vi "PvgeneratorOP150_2.vi"(8 "errin":errorcluster, 9 "BDD":T1, 10 "network":path, 11 "path in":path) -> (0 "sortie d'erreur":errorcluster caption="errout", 1 "network out":path, 2 "tout bon":bool, 3 "Chaîne":string)   [LabVIEW 2020]
uses:
  OP150/VG/IS30%.vi
  OP150/VG/PN.vi
  <vilib>/Utility/config.llb/NI_LVConfig.lvlib
  OP150 - Copie/SubVI/VG_HYDRAU.vi
panel:
  out "nombre de remplacements":i32
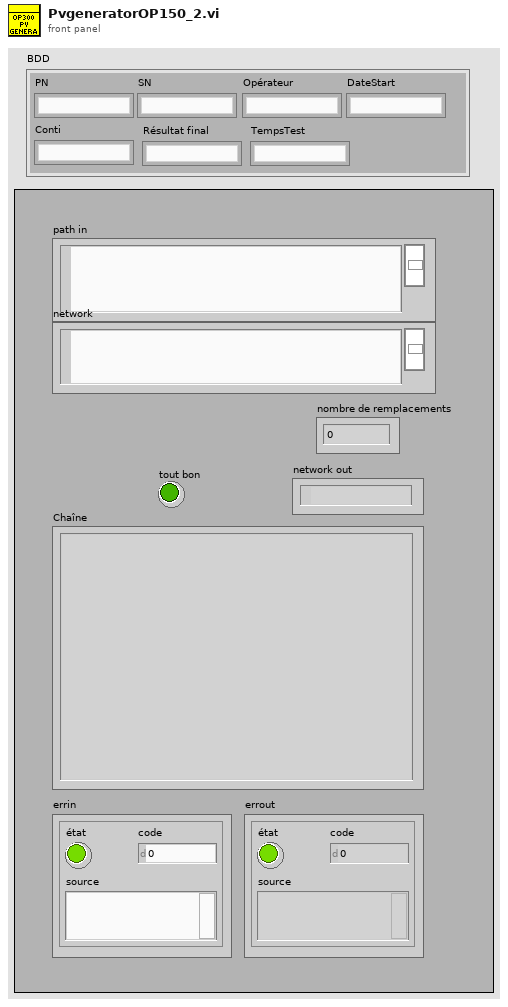
[diagram p1: front panel]
types:
  T1 = cluster{"PN":string, "Opérateur":string, "Conti":string, "Résultat final":string, "SN":string, "DateStart":string, "TempsTest":string}
  T2 = enum16{"open", "replace", "create", "open or create", "replace or create", "replace or create with confirmation"}
  T3 = typedef "NI_LVConfig.lvlib/Config Data RefNum.ctl" = refnum<k1>
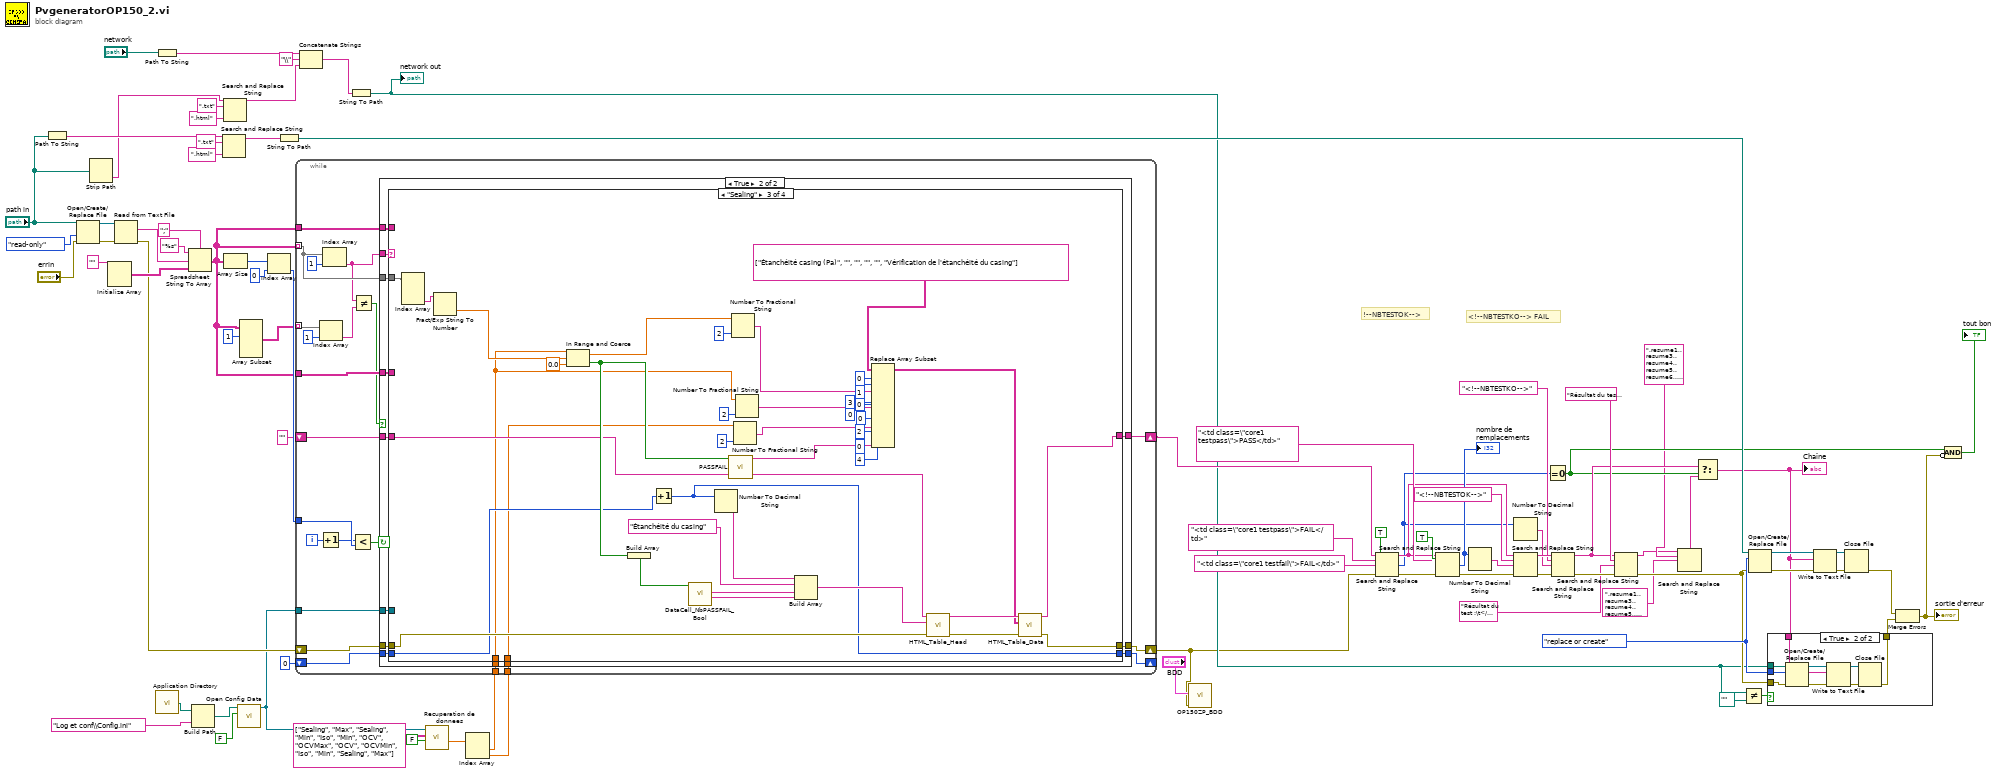
[diagram p0: block diagram]
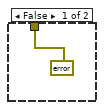
[diagram p2: hidden frame]
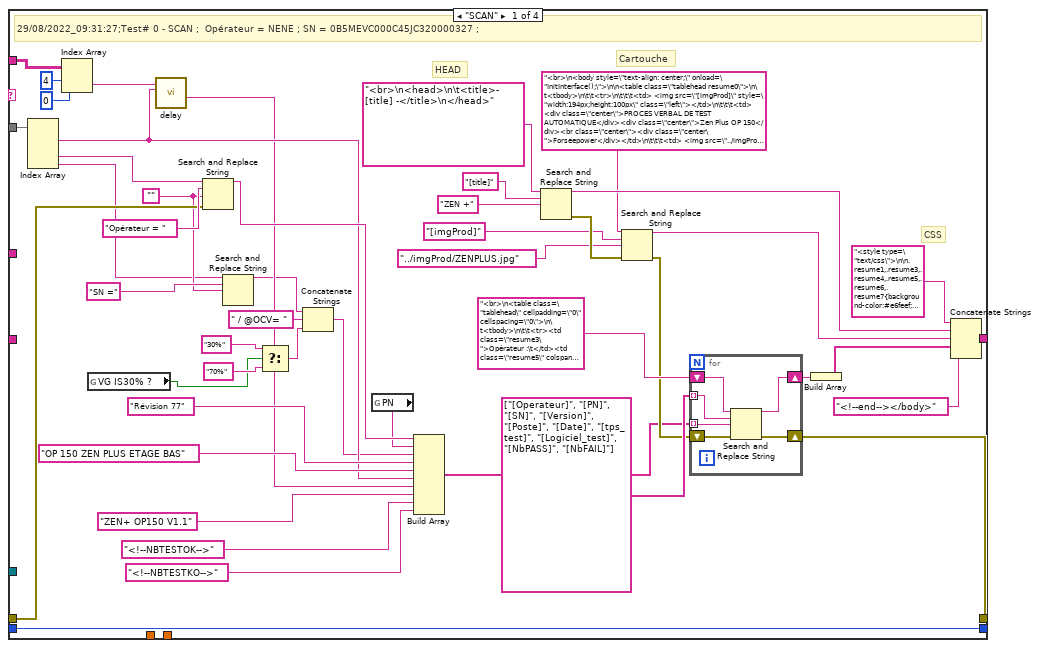
[diagram p4: hidden frame]
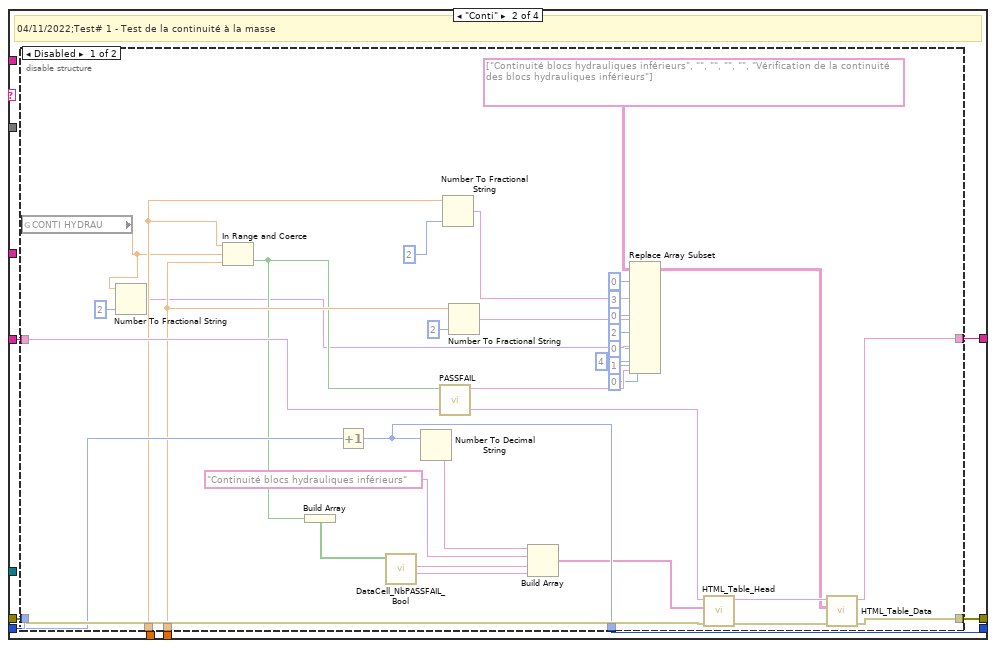
[diagram p5: hidden frame]
diagram:
  w44 = T2."replace or create" ("opération (0 : open)")
  # "<!--NBTESTKO--> FAIL"
  # "!--NBTESTOK-->"
  n1 = Path To String(path="path in") -> (string=w65:string)
  n2 = Open/Create/Replace File(file path (use dialog)="path in", error in="errin", access (0:read/write)=enum16{"read/write", "read-only", "write-only"}."read-only" ("accès (0 : read/write)")) -> (refnum out=w66:refnum<file>, error out=w83:errorcluster)  [unwired: 3 in, 1 out]
  n3 = Strip Path(path="path in") -> (name=w25:string)  [unwired: 1 out]
  n4 = Initialize Array("") -> (w81:string[][])  [unwired: 2 in]
  n5 = Read from Text File(file (use dialog)=w66, error in=w83) -> (text=w79:string, error out=w71:errorcluster)  [unwired: 2 in, 2 out]
  n6 = Path To String(path="network") -> (string=w24:string)
  n7 = call <vilib>:"Application Directory.vi"() -> ("Application Directory"=w16:path)
  n8 = Spreadsheet String To Array(delimiter (Tab)=";" ("séparateur (Tabulation)"), format string="%s" ("chaîne de format"), spreadsheet string=w79, array type (2D Dbl)=w81) -> (array=w6:string[][])
  n9 = Build Path(base path=w16, name or relative path="Log et conf\\Config.ini") -> (appended path=w19:path)
  n10 = Search and Replace String(input string=w65, search string=".txt" ("chaîne recherchée"), replace string=".html" ("chaîne de remplacement (\"\")")) -> (result string=w62:string)  [unwired: 5 in, 3 out]
  n11 = Search and Replace String(input string=w25, search string=".txt" ("chaîne recherchée"), replace string=".html" ("chaîne de remplacement (\"\")")) -> (result string=w22:string)  [unwired: 5 in, 3 out]
  n12 = Array Size(array=w6) -> (size(s)=w77:i32[])
  n13 = call <vilib>:"Open Config Data.vi"("create file if necessary (T)"=FALSE, "configuration file path"=w19) -> ("refnum"=w3:T3)  [unwired: 7 in, 2 out]
  n14 = Array Subset(array=w6, index (row)=1 ("indice")) -> (w4:string[][])  [unwired: 3 in]
  n15 = Index Array(array=w77, index=0 ("indice")) -> (element=w75:i32)
  n16 = String To Path(string=w62) -> (path=w61:path)
  n17 = Concatenate Strings(w24, "\\" ("chaîne"), w22) -> (w21:string)
  n18 = String To Path(string=w21) -> (path=w27:path)
  "network out" <- w27
  n19 = call "Recuperation de donnees.vi"("Est-ce un string?"=FALSE, "Array in"=string[][] [["Sealing", "Max"], ["Sealing", "Min"], ["Iso", "Min"], ["OCV", "OCVMax"], ["OCV", "OCVMin"], ["Iso", "Min"], ["Sealing", "Max"]], "Refnum in"=w3) -> ("Array"=w13:dbl[])  [unwired: 7 in, 1 out]
  n20 = Index Array(array=w13) -> (element #1=w12:dbl, element #2=w11:dbl)  [unwired: 2 in]
  n21 = while {
    tunnel: w75 -> [w105]
    tunnel: w6 -> [w102] mode=indexing
    shift-right: [w101] -> w1
    shift-left: w71 -> [w100]
    shift-right: [w94] -> w60
    shift-left: "" -> [w99]
    shift-right: [w97] -> _
    shift-left: 0 -> [w98]
    tunnel: w6 -> [w96]
    tunnel: w12 -> [w93]
    tunnel: w11 -> [w92]
    tunnel: w6 -> [w91]
    tunnel: w4 -> [w89] mode=indexing
    tunnel: w3 -> [w85]
    i -> [w106]
    stop <- w104 continue-if-true
    n22 = Index Array(array=w89, index=1 ("indice")) -> (element=w88:string)
    n23 = Increment(x=w106) -> (x+1=w95:i32)
    n24 = Index Array(array=w102, index=1 ("indice")) -> (element=w87:string)
    n25 = Less?(x=w95, y=w105) -> (x < y?=w104:bool)
    n26 = Not Equal?(x=w87, y=w88) -> (x != y?=w86:bool)
    n27 = case shown="True" w86 {
      tunnel: w102 -> [_ w122]
      tunnel: [w108 w121] -> w101
      tunnel: w100 -> [w108 w120]
      tunnel: w99 -> [w109 w119]
      tunnel: w98 -> [w107 w118]
      tunnel: [w107 w117] -> w97
      tunnel: w96 -> [_ w116]
      tunnel: [w109 w115] -> w94
      tunnel: w87 -> [_ w114]
      tunnel: w93 -> [_ w113]
      tunnel: w92 -> [_ w112]
      tunnel: w91 -> [_ w111]
      tunnel: w85 -> [_ w110]
      frame False {
      }
      frame True {
        n28 = case shown="\"Sealing\"" w114 {
          tunnel: w120 -> [w167 w183 w240 w260]
          tunnel: w122 -> [w169 _ w221 _]
          tunnel: [w146 w182 w239 w260] -> w121
          tunnel: w119 -> [_ w181 w235 w258]
          tunnel: w118 -> [w145 w180 w238 w259]
          tunnel: [w145 w179 w237 w259] -> w117
          tunnel: w116 -> [_ _ _ _]
          tunnel: [w144 w178 w236 w258] -> w115
          tunnel: w113 -> [_ w177 w232 _]
          tunnel: w112 -> [_ w176 w228 _]
          tunnel: w111 -> [w137 _ _ _]
          tunnel: w110 -> [_ _ _ _]
          frame "SCAN" {
            w140 = ""
            # "Cartouche"
            # "HEAD"
            # "CSS"
            # "29/08/2022_09:31:27;Test# 0 - SCAN ;  Opérateur = NENE ; SN = 0B5MEVC000C45JC320000327 ;"
            n29 = Index Array(array=w169) -> (element #1=w133:string, element #3=w143:string, element #4=w138:string)  [unwired: 4 in, 1 out]
            n30 = Index Array(array=w137, index (row)=4, index (col)=0 ("disabled index (col)")) -> (element=w134:string)
            n31 = global read "IS30%.vi" "VG IS30% ?"() -> (w124:bool)
            n32 = call "delay.vi"("String"=w133, "String 2"=w134) -> ("Delay calculé"=w132:string)  [unwired: 9 in]
            n33 = Search and Replace String(input string=w143, search string="Opérateur = " ("chaîne recherchée"), replace string=w140, error in=w167) -> (result string=w142:string)  [unwired: 4 in, 3 out]
            n34 = Search and Replace String(input string=w138, search string="SN =" ("chaîne recherchée"), replace string=w140) -> (result string=w130:string)  [unwired: 5 in, 3 out]
            n35 = Select(t="30%" ("y"), s=w124, f="70%" ("y")) -> (s? t:f=w127:string)
            n36 = Concatenate Strings(w130, " / @OCV= " ("chaîne"), w127) -> (w129:string)
            n37 = global read "PN.vi" "PN"() -> (w123:string)
            n38 = Build Array(w142, w123, w129, "Révision 77" ("element"), "OP 150 ZEN PLUS ETAGE BAS" ("chaîne"), w133, w132, "ZEN+ OP150 V1.1" ("chaîne"), "<!--NBTESTOK-->" ("chaîne"), "<!--NBTESTKO-->" ("chaîne")) -> (w147:string[])
            n39 = Search and Replace String(input string="<br>\n<head>\n\t<title>- [title] -</title>\n</head>", search string="[title]" ("chaîne recherchée"), replace string="ZEN +" ("Title")) -> (result string=w163:string, error out=w162:errorcluster)  [unwired: 5 in, 2 out]
            n40 = Search and Replace String(input string="<br>\n<body style=\"text-align: center;\" onload=\"InitInterface();\">\n\n<table class=\"tablehead resume0\">\n\t<tbody>\n\t\t<tr>\n\t\t\t<td> <img src=\"[imgProd]\" style=\"width:194px;height:100px\" class=\"left\"></td>\n\t\t\t<td> <div class=\"center\">PROCES VERBAL DE TEST AUTOMATIQUE</div><div class=\"center\">Zen Plus OP 150</div><br class=\"center\"><div class=\"center\">Forseepower</div></td>\n\t\t\t<td> <img src=\"../imgProd/LOGO FORSEE.png\" style=\"width:auto;height:auto\"  class=\"right\"></td>\n\t\t</tr>\n\t</tbody>\n</table>", search string="[imgProd]", replace string="../imgProd/ZENPLUS.jpg" ("imgProd"), error in=w162) -> (result string=w160:string, error out=w157:errorcluster)  [unwired: 4 in, 2 out]
            n41 = for {
              shift-right: [w174] -> w156
              shift-left: "<br>\n<table class=\"tablehead\" cellpadding=\"0\" cellspacing=\"0\">\n\t<tbody>\n\t\t<tr><td class=\"resume3\">Opérateur :\t</td><td class=\"resume5\" colspan=\"3\">[Operateur]</td></tr>\n\t\t<tr><td class=\"resume3\">PN : </td><td class=\"resume5\" colspan=\"3\">[PN]</td></tr>\n\t\t<tr><td class=\"resume3\">SN : </td><td class=\"resume5\" colspan=\"3\">[SN]</td></tr>\n\t\t<tr><td class=\"resume3\">Version : </td><td class=\"resume5\" colspan=\"3\">[Version]</td></tr>\n\t\t<tr><td class=\"resume3\">Poste : </td><td class=\"resume5\" colspan=\"3\">[Poste]</td></tr>\t\t\n\t\t<tr><td class=\"resume3\">Date du test : </td><td class=\"resume5\" colspan=\"3\">[Date]</td></tr>\n\t\t<tr><td class=\"resume3\">Temps de test : </td><td class=\"resume5\" colspan=\"3\">[tps_test]</td></tr>\n\t\t<tr><td class=\"resume3\">Logiciel de test :\t</td><td class=\"resume5\" colspan=\"3\">[Logiciel_test]</td></tr>\n\t\t<tr><td class=\"resume3\">Résultat du test :\t</td><td class=\"resume5\" colspan=\"3\"><div><span style=\"float:left\" id=\"result\"><font size = \"5pt\" color=\"green\"><b>CONFORME</b></font><b><font size = \"5pt\"> ( </font><font size = \"5pt\" color=\"green\">[NbPASS] PASS </font>  <font size = \"5pt\"> / </font><font size = \"5pt\" color=\"red\">[NbFAIL] FAIL</font> <font size = \"5pt\"> ) </font></b></span></div></td></tr>\n\t</tbody>\n</table>" -> [w175]
              tunnel: string[] ["[Operateur]", "[PN]", "[SN]", "[Version]", "[Poste]", "[Date]", "[tps_test]", "[Logiciel_test]", "[NbPASS]", "[NbFAIL]"] -> [w171] mode=indexing
              tunnel: w147 -> [w170] mode=indexing
              shift-right: [w172] -> w146
              shift-left: w157 -> [w173]
              n42 = Search and Replace String(input string=w175, search string=w171, replace string=w170, error in=w173) -> (result string=w174:string, error out=w172:errorcluster)  [unwired: 4 in, 2 out]
            }
            n43 = Build Array(w156) -> (w155:string[])
            n44 = Concatenate Strings("<style type=\"text/css\">\n\n.resume1,.resume3,.resume4,.resume5,.resume6,.resume7{background-color:#e6feef;padding:7px;border:1px solid black;}\n.resume0{border:1px solid black;background-color:#e6feef;font-weight: bold;padding:0px;text-align: center;}\n.resume1{width:350px;text-align:right;font-weight:bold;}\n.resume3{width:350px;text-align:right;border-top:0px solid black;font-weight:bold;}\n.resume4{border-left:0px solid black;width:290px;}\n.resume5{width:290px;border-left:0px solid black;border-top:0px solid black;}\n.resume6{border-left:0px solid black;width:60px;}\n.resume7{border-left:0px solid black;border-top:0px solid black;width:60px;}\n.title1{text-align: left;background-color:#e6f4fe;padding:10px;border:1px solid #101010;}\n.title2{width: 30px;text-align: center;background-color:#e6f4fe;padding:1px;border:1px solid #101010;border-left:0px solid black;font-weight: bold;}\n.title2 a:link{text-decoration:none;}\n.entete0,.entete1,.entete2,.time2{text-align: center;background-color:#feeec9;padding:7px;border:1px solid black;font-weight: bold;}\n.entete0{width:45px;border-right:0px solid black;}\n.entete1{width:505px;}\n.entete2{width:95px;border-right:0px solid black;}\n.time2{border-left:0px solid black;width:145px;font-size:11px;}\n.core0,.core1,.core2,.core3,.core4,.time{text-align: center;background-color:#fafed3;padding:7px;border:1px solid black;}\n.core0, .core1,.core3,.core4{width:95px;border-top:0px solid black;border-right:0px solid black;}\n.core0{width:45px;}\n.core2{border-top:0px solid black;width:505px;}\n.core3{width:200px;}\n.core4{width:300px;}\n.time{width:145px;border-top:0px solid black;border-left:0px solid black;font-size:11px;}\n.false .core0,.false .core1,.false .core2,.false .core3,.false .core4,.false .time{background-color:#f4f4f4;}\n.false .entete0,.false .entete1,.false .entete2,.false .time2{background-color:#dadada;}\n.false .title1,.false .title2,.false .resultentete .testpass,.false .resultentete .testfail,.false .resultentete .testtime{background-color:#c5cac9;color: blue;}\n.false .title2 a:link{text-decoration:none;color: blue;}\n.comment1,.comment2,.time3{width: 890px;background-color:#e9e8e9;padding:7px;border:1px solid black;border-top:0px solid black;text-align:left;}\n.comment2{border-right:0px solid black;width: 45px;text-align: center;}\n.time3{width: 145px;border-left:0px solid black;font-size:11px;}\n.fixe1{background: -moz-linear-gradient(center top , #101010 10%, #555555 80%) repeat scroll 0 0 transparent;background: -webkit-gradient(linear, left top, left bottom, from(#101010), to(#555555));border:2px solid orange;position : fixed;margin-top:20px;display:none;overflow-y:scroll;max-height:350px;text-shadow: 0px 0px 0 #333333;text-align:left;font-size:10px;padding:10px;margin-left:-162px;border-radius: 15px 15px 15px 15px;}\n.menufixe, .menufixelock{background: -moz-linear-gradient(center top , #101010 80%, transparent 20%) repeat scroll 0 0 transparent;background: -webkit-gradient(linear, left top, left bottom, from(#101010), color-stop(0.65, #101010), to(transparent)) repeat scroll 0 0 transparent;margin: -52px 0px 0px -9px;width:100%;position:fixed;height:55px;-moz-transition: margin 1s;-webkit-transition: margin 1s;}\n.menufixelock, .menufixe:hover{margin: -9px 0px 0px -9px;}\n.lockmenu, .separation,.separationmenu{text-align:center;background: -moz-linear-gradient(center top , #555555 10%, #111111 80%) repeat scroll 0 0 transparent;background: -webkit-gradient(linear, left top, left bottom, from(#555555), to(#111111));border: 1px solid white;border-radius: 10px 10px 10px 10px;box-shadow: 0 -1px 1px #555555 inset;color: #999999;font-weight: bold;width: 100px;padding: 2px;text-decoration: none;}\n.tablehead{width: 1000px;font-family: Verdana;font-size: 12px;margin-left: auto;margin-right: auto;}\n.tablenull{font-family: Verdana;font-size: 11px;margin-left: auto;margin-right: auto;}\n.separationmenu:hover div{display: inline;}\n.lockmenu:hover, .separation:hover,.separationmenu:hover{border: 1px solid orange;cursor:pointer;}\n.lockmenu:hover{border: 1px solid red;cursor:pointer;}\n.separationright{padding:10px;}\ndiv a:link{text-decoration:none;color:#cbcbcb;}\ndiv a:hover{text-decoration:underline;color:#cbcbcb;}\nspan a:link{text-decoration:none;color:#cbcbcb;}\nspan a:hover{text-decoration:none;color:#cbcbcb;}\n.false{color: blue;}\n.testpass{color: green;font-weight: bold;}\n.testfail{color: red;font-weight: bold;}\n.testtime{color: blue;font-weight: bold;}\n.resultentete{font-weight: bold;font-size: 11px;min-width: 200px;text-align:right;}\n.infohard{border: 1px solid black;background-color: white;text-align: center;width: 16px;height: 16px;border-radius: 5px;font-weight: bold;box-shadow: 0 -1px 2px #555555 inset;}\n.infohard:hover{background-color:#feeec9;cursor:pointer;}\n.footerhard{padding-top:30px;}\n.confighard{font-size:10px;width:110px;}\n.circlemain{margin-left:auto;margin-right:auto;}\n.circletext,.circleform{padding-top: 3px;text-align:center;font-size: 10px;width:200px;}\n.circleform{padding-bottom: 3px;padding-top: 1px;}\n.circle{border: 1px solid black;border-collapse: collapse;border-radius: 15px;box-shadow: 1px 1px 0 #505050;height: 15px;width: 15px;display:inline-block;}\n.bookmarkon, .bookmarkoff{background-color: yellow;border: 1px solid black;border-collapse: collapse;border-radius: 10px 10px 10px 10px;box-shadow: 1px 1px 0 #505050;height: 12px;width: 12px;position: absolute;margin-left:22px;cursor: help;}\n.bookmarkoff{background-color: transparent;border: 1px solid #CECECE;box-shadow: none;cursor: copy;}\n.false .bookmarkoff{background-color: transparent;border: 1px solid #E6E1E1;box-shadow: none;cursor: copy;}\n.bookmarkmaster{height: 15px;margin-right: 12px;width: 60px;}\n.bookmarkmaster:hover .bookmarkprev,.bookmarkmaster:hover .bookmarksuiv{display:block;}\n.bookmarkprev, .bookmarksuiv {cursor: pointer;font-size: 25px;font-weight: bold;margin-top: -10px;position: absolute;display:none;}\n.bookmarkprev{margin-left: 2px;}\n.bookmarksuiv{margin-left: 43px;}\n.plus, .moins{background-color: #F4F4F4;border: 1px solid #848484;border-radius: 20px;color: #848484;font-family: arial;font-size: 16px;font-weight: bold;height: 20px;margin-left: 4px;text-align: center;width: 20px;}\n.moins{font-size: 15px;}\n.plus:hover, .moins:hover{background-color: #DADADA;border: 1px solid black;color: black;cursor:pointer;}\n.backtothetop {position: fixed; right: 50%; margin-right: -555px; bottom: 10px; font-size: 35px; font-weight: bold; border: 1px solid #7D7B91; width: 40px; height: 40px; line-height:52px; text-align: center;border-radius: 8px; opacity: 0.25; background-color: #F5F5F5; color:#7D7B91;}\n.backtothetop:hover {opacity: 1; cursor:pointer;}\n.libversion {font-size: 8px;font-weight: normal;padding-right: 10px;text-align: right;}\n.lockmenu {width: 18px;font-size: 12px;}\n.left {display: block; margin-left: 1px;margin-right: auto;}\n.right {display: block; margin-right: 1px;margin-left: auto;}\n.center {display: block; margin-left: auto;margin-right: auto;}\n\n</style>", w163, w160, w155, "<!--end--></body>") -> (w144:string)
          }
          frame "Conti" {
            # "04/11/2022;Test# 1 - Test de la continuité à la masse"
            n45 = disable-structure shown="Disabled" {
              disable-tunnel: w183 -> [w218 _]
              disable-tunnel: [w217 _] -> w182
              disable-tunnel: w181 -> [w216 _]
              disable-tunnel: w180 -> [w215 _]
              disable-tunnel: [w214 _] -> w179
              disable-tunnel: [w213 _] -> w178
              disable-tunnel: w177 -> [w212 _]
              disable-tunnel: w176 -> [w211 _]
              frame Disabled {
                n46 = global read "VG_HYDRAU.vi" "CONTI HYDRAU"() -> (w197:dbl)
                n47 = Number To Fractional String(number=w197, precision (6)=i16 2 ("précision (6)")) -> (F-format string=w189:string)  [unwired: 2 in]
                n48 = In Range and Coerce(upper limit=w212, x=w197, lower limit=w211) -> (In Range?=w198:bool)  [unwired: 1 out]
                n49 = Build Array(w198) -> (w203:bool[])
                n50 = Increment(x=w215) -> (x+1=w214:i32)
                n51 = call "DataCell_NbPASSFAIL_Bool.vi"("Tableau en entrée"=w203) -> ("Chaîne"=w201:string, "Chaîne 2"=w202:string)  [unwired: 8 in, 1 out]
                n52 = Number To Decimal String(number=w214) -> (decimal integer string=w206:string)  [unwired: 1 in]
                n53 = call "PASSFAIL.vi"("E"=w198) -> ("S"=w186:string)  [unwired: 10 in]
                n54 = Number To Fractional String(number=w212, precision (6)=i16 2) -> (F-format string=w195:string)  [unwired: 2 in]
                n55 = Number To Fractional String(number=w211, precision (6)=i16 2) -> (F-format string=w192:string)  [unwired: 2 in]
                n56 = Build Array(w206, "Continuité blocs hydrauliques inférieurs" ("élément"), w202, w201) -> (w209:string[])
                n57 = Replace Array Subset(array=string[][] [["Continuité blocs hydrauliques inférieurs", "", "", "", "", "Vérification de la continuité des blocs hydrauliques inférieurs"]] ("Tableau"), new element #1=w195, index (row) #1=0 ("indice (ligne)"), index (col) #1=3 ("indice désactivé (col)"), new element #2=w192, index (row) #2=0 ("indice (ligne)"), index (col) #2=2 ("indice désactivé (col)"), new element #3=w189, index (row) #3=0 ("indice (ligne)"), index (col) #3=1 ("indice désactivé (col)"), new element #4=w186, index (row) #4=0 ("indice (ligne)"), index (col) #4=4 ("indice désactivé (col)")) -> (w204:string[][])
                n58 = call "HTML_Table_Head.vi"("entrée d'erreur (pas d'erreur)"=w218, "Tableau"=w209, "chaîne en entrée"=w216) -> ("sortie d'erreur"=w208:errorcluster, "result string"=w207:string)  [unwired: 7 in]
                n59 = call "HTML_Table_Data.vi"("entrée d'erreur (pas d'erreur)"=w208, "Tableau"=w204, "chaîne en entrée"=w207) -> ("sortie d'erreur"=w217:errorcluster, "result string"=w213:string)  [unwired: 7 in]
              }
              frame Enabled {
              }
            }
          }
          frame "Sealing" {
            (unwired) 0 ("index (row)")
            n60 = Index Array(array=w221) -> (element #3=w220:string)  [unwired: 3 in, 2 out]
            n61 = Fract/Exp String To Number(string=w220) -> (number=w233:dbl)  [unwired: 3 in, 1 out]
            n62 = In Range and Coerce(upper limit=w232, x=w233, lower limit=0.0) -> (coerced(x)=w234:dbl, In Range?=w246:bool)
            n63 = Build Array(w246) -> (w251:bool[])
            n64 = Increment(x=w238) -> (x+1=w237:i32)
            n65 = call "DataCell_NbPASSFAIL_Bool.vi"("Tableau en entrée"=w251) -> ("Chaîne"=w249:string, "Chaîne 2"=w250:string)  [unwired: 8 in, 1 out]
            n66 = Number To Decimal String(number=w237) -> (decimal integer string=w254:string)  [unwired: 1 in]
            n67 = call "PASSFAIL.vi"("E"=w246) -> ("S"=w224:string)  [unwired: 10 in]
            n68 = Number To Fractional String(number=w234, precision (6)=i16 2) -> (F-format string=w245:string)  [unwired: 2 in]
            n69 = Number To Fractional String(number=w228, precision (6)=i16 2) -> (F-format string=w227:string)  [unwired: 2 in]
            n70 = Number To Fractional String(number=w232, precision (6)=i16 2) -> (F-format string=w242:string)  [unwired: 2 in]
            n71 = Build Array(w254, "Étanchéité du casing" ("élément"), w250, w249) -> (w257:string[])
            n72 = Replace Array Subset(array=string[][] [["Étanchéité casing (Pa)", "", "", "", "", "Vérification de l'étanchéité du casing"]] ("Tableau"), new element #1=w245, index (row) #1=0 ("indice (ligne)"), index (col) #1=1 ("indice désactivé (col)"), new element #2=w242, index (row) #2=0 ("index (row)"), index (col) #2=3 ("disabled index (col)"), new element #3=w227, index (row) #3=0 ("index (row)"), index (col) #3=2 ("disabled index (col)"), new element #4=w224, index (row) #4=0 ("index (row)"), index (col) #4=4 ("disabled index (col)")) -> (w252:string[][])
            n73 = call "HTML_Table_Head.vi"("entrée d'erreur (pas d'erreur)"=w240, "Tableau"=w257, "chaîne en entrée"=w235) -> ("sortie d'erreur"=w256:errorcluster, "result string"=w255:string)  [unwired: 7 in]
            n74 = call "HTML_Table_Data.vi"("entrée d'erreur (pas d'erreur)"=w256, "Tableau"=w252, "chaîne en entrée"=w255) -> ("sortie d'erreur"=w239:errorcluster, "result string"=w236:string)  [unwired: 7 in]
          }
          frame "NULL", Default {
            # "NULL"
          }
        }
      }
    }
  }
  n75 = call "OP150ZP_BDD.vi"("errin"=w1, "DATA IN"="BDD") -> ()  [unwired: 9 in, 1 out]
  n76 = Search and Replace String(replace all?=TRUE ("tout remplacer ? (F)"), input string=w60, search string="<td class=\"core1 testpass\">FAIL</td>" ("chaîne recherchée"), replace string="<td class=\"core1 testfail\">FAIL</td>" ("chaîne de remplacement (\"\")"), error in=w1) -> (result string=w45:string, number of replacements=w40:i32, error out=w56:errorcluster)  [unwired: 3 in, 1 out]
  n77 = Search and Replace String(replace all?=TRUE ("tout remplacer ? (F)"), input string=w45, search string="<td class=\"core1 testpass\">PASS</td>" ("chaîne recherchée"), error in=w56) -> (number of replacements=w48:i32, error out=w52:errorcluster)  [unwired: 4 in, 2 out]
  "nombre de remplacements" <- w48
  n78 = Number To Decimal String(number=w48) -> (decimal integer string=w47:string)  [unwired: 1 in]
  n79 = Number To Decimal String(number=w40) -> (decimal integer string=w46:string)  [unwired: 1 in]
  n80 = Search and Replace String(input string=w45, search string="<!--NBTESTOK-->" ("chaîne recherchée"), replace string=w47, error in=w52) -> (result string=w53:string, error out=w51:errorcluster)  [unwired: 4 in, 2 out]
  n81 = Equal To 0?(x=w40) -> (x = 0?=w32:bool)
  n82 = Search and Replace String(input string=w53, search string="<!--NBTESTKO-->" ("chaîne recherchée"), replace string=w46, error in=w51) -> (result string=w35:string, error out=w39:errorcluster)  [unwired: 4 in, 2 out]
  n83 = Search and Replace String(input string=w35, search string="Résultat du test :\t</td><td class=\"resume5\" colspan=\"3\"><div><span style=\"float:left\" id=\"result\"><font size = \"5pt\" color=\"green\"><b>CONFORME</b>", replace string="Résultat du test :\t</td><td class=\"resume5\" colspan=\"3\"><div><span style=\"float:left\" id=\"result\"><font  size = \"5pt\" color=\"red\"><b>NON CONFORME</b>", error in=w39) -> (result string=w8:string, error out=w38:errorcluster)  [unwired: 4 in, 2 out]
  n84 = Search and Replace String(input string=w8, search string=".resume1,.resume3,.resume4,.resume5,.resume6,.resume7{background-color:#e6feef;padding:7px;border:1px solid black;}\n.resume0{border:1px solid black;background-color:#e6feef;font-weight: bold;padding:0px;text-align: center;}", replace string=".resume1,.resume3,.resume4,.resume5,.resume6,.resume7{background-color:#fdebd0;padding:7px;border:1px solid black;}\n.resume0{border:1px solid black;background-color:#fdebd0;font-weight: bold;padding:0px;text-align: center;}") -> (result string=w7:string)  [unwired: 5 in, 3 out]
  n85 = Select(t=w35, s=w32, f=w7) -> (s? t:f=w36:string)
  "Chaîne" <- w36
  n86 = Not Equal?(x=w27, y=path "") -> (x != y?=w29:bool)
  n87 = Open/Create/Replace File(file path (use dialog)=w61, error in=w38, operation (0:open)=w44) -> (refnum out=w67:refnum<file>, error out=w69:errorcluster)  [unwired: 3 in, 1 out]
  n88 = case shown="True" w29 {
    tunnel: w44 -> [_ w266]
    tunnel: w27 -> [_ w265]
    tunnel: w38 -> [_ w264]
    tunnel: w36 -> [_ w263]
    tunnel: [errorcluster {"status"=FALSE, "code"=0, "source"=""} ("error out") w262] -> w34
    frame False {
    }
    frame True {
      n89 = Open/Create/Replace File(file path (use dialog)=w265, error in=w264, operation (0:open)=w266) -> (refnum out=w267:refnum<file>, error out=w269:errorcluster)  [unwired: 3 in, 1 out]
      n90 = Write to Text File(file (use dialog)=w267, text=w263, error in=w269) -> (refnum out=w268:refnum<file>, error out=w270:errorcluster)  [unwired: 1 in, 1 out]
      n91 = Close File(refnum=w268, error in=w270) -> (error out=w262:errorcluster)  [unwired: 1 out]
    }
  }
  n92 = Write to Text File(file (use dialog)=w67, text=w36, error in=w69) -> (refnum out=w68:refnum<file>, error out=w70:errorcluster)  [unwired: 1 in, 1 out]
  n93 = Close File(refnum=w68, error in=w70) -> (error out=w33:errorcluster)  [unwired: 1 out]
  n94 = Merge Errors(w33, w34) -> (w31:errorcluster)
  "sortie d'erreur" <- w31
  n95 = Compound Arithmetic op=AND ("Opérateur arithmétique")(w32, invert w31) -> (→"tout bon":bool)
